vi "Add Instrument Group to Tree.vi"(7 "ItemType":T1=enum."Temp Group", 8 "error in (no error)":errorcluster, 9 "#ofComparators (New ComparatorID)":i32, 10 "Comparator Tag (Parent)":string, 11 "TreeControl in":refnum<vi>) -> (0 "error out":errorcluster, 2 "Instrument Group Tag out":string, 3 "TreeControl out":refnum<vi>)   [LabVIEW 2018]
uses:
  TypeDefs/Tree Item Type.ctl
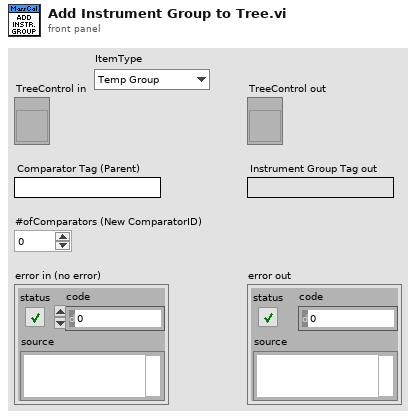
[diagram p1: front panel]
types:
  T1 = typedef "Tree Item Type.ctl" = enum16{"Comparator", "Temp Group", "Press Group", "Hygro Group", "Thermometer", "PressureTransducer", "Hygrometers", "Add Comparator", "Add Thermometer", "Add Barometer", "Add Hygrometer"}
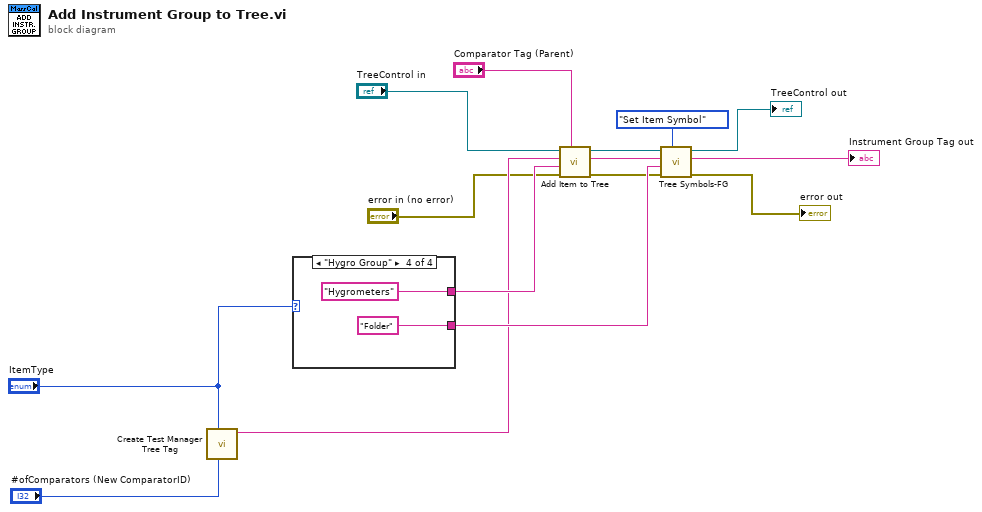
[diagram p0: block diagram]
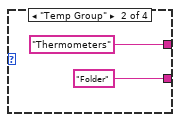
[diagram p3: hidden frame]
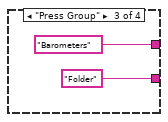
[diagram p4: hidden frame]
diagram:
  n1 = call "Create Test Manager Tree Tag.vi"("Comparator ID"="#ofComparators (New ComparatorID)", "ItemType"="ItemType") -> ("Tag"=w5:string)  [unwired: 7 in, 2 out]
  n2 = case shown="\"Hygro Group\"" "ItemType" {
    tunnel: [_ "Folder" ("Symbol Name") "Folder" ("Symbol Name") "Folder" ("Symbol Name")] -> w10
    tunnel: [_ "Thermometers" ("Item Name") "Barometers" ("Item Name") "Hygrometers" ("Item Name")] -> w6
    frame "Comparator", Default {
    }
    frame "Temp Group" {
    }
    frame "Press Group" {
    }
    frame "Hygro Group" {
    }
  }
  n3 = call "Add Item to Tree.vi"("Parent Tag"="Comparator Tag (Parent)", "error in (no error)"="error in (no error)", "Item Name"=w6, "Item Tag"=w5, "Tree Ref"="TreeControl in") -> ("error out"=w3:errorcluster, "Item Tag out"=w9:string, "reference out"=w8:refnum<vi>)  [unwired: 3 in, 1 out]
  n4 = call "Tree Symbols-FG.vi"("Actions"=enum16{"Init Symbols", "Set Item Symbol"}."Set Item Symbol", "error in (no error)"=w3, "Symbol Name"=w10, "Item Tag"=w9, "Tree Ref"=w8) -> ("error out"=→"error out":errorcluster, "Item Tag out"=→"Instrument Group Tag out":string, "Tree Ref out"=→"TreeControl out":refnum<vi>)  [unwired: 4 in]
